vi "Save MES errors.vi"(9 "Sent parameters":variant, 10 "Error Text":string, 11 "Operation":string) -> ()   [LabVIEW 2023]
uses:
  <vilib>/Utility/file.llb/Write Delimited Spreadsheet (string).vi
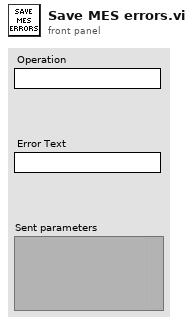
[diagram p1: front panel]
types:
  T1 = cluster{"MaterialCode":string, "Operator":string, "SerialNo":string}
  T2 = cluster{"HuNo":string, "MaterialCode":string, "Mode":i32, "Operator":string, "PackingInstructions":string, "ProductionVersion":string, "SerialNo":string}
  T3 = cluster{"EquipmentCode":string, "Mode":i32, "Operator":string}
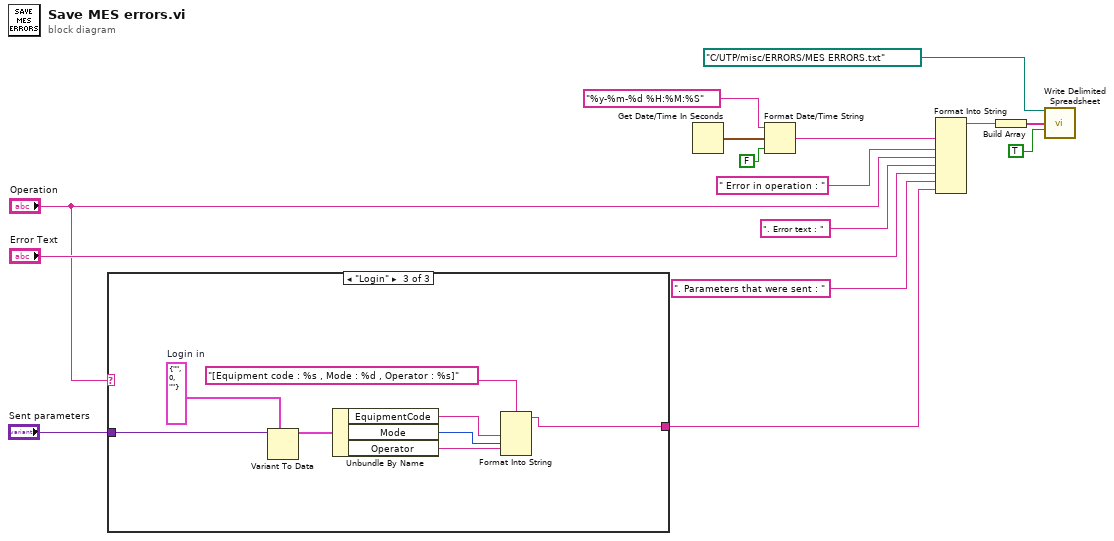
[diagram p0: block diagram]
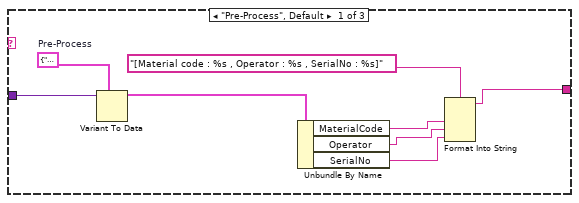
[diagram p2: hidden frame]
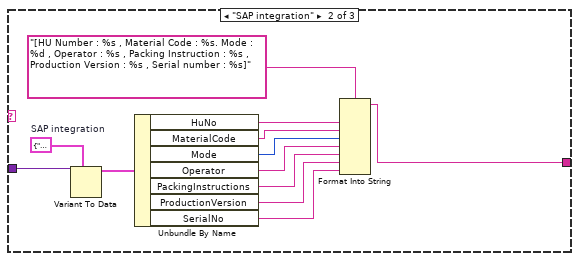
[diagram p3: hidden frame]
diagram:
  n1 = case shown="\"Login\"" "Operation" {
    tunnel: "Sent parameters" -> [w16 w35 w43]
    tunnel: [w18 w25 w36] -> w1
    frame "Pre-Process", Default {
      w17 = T1 {"MaterialCode"="", "Operator"="", "SerialNo"=""}  # Pre-Process
      n2 = Variant To Data(type=w17, Variant=w16) -> (data=w20:T1)  [unwired: 1 in, 1 out]
      n3 = Unbundle By Name(w20) -> ("MaterialCode"=w21:string, "Operator"=w22:string, "SerialNo"=w23:string)
      n4 = Format Into String(format string="[Material code : %s , Operator : %s , SerialNo : %s]", w21, w22, w23) -> (resulting string=w18:string)  [unwired: 2 in, 1 out]
    }
    frame "SAP integration" {
      w34 = T2 {"HuNo"="", "MaterialCode"="", "Mode"=0, "Operator"="", "PackingInstructions"="", "ProductionVersion"="", "SerialNo"=""}  # SAP integration
      n5 = Variant To Data(type=w34, Variant=w35) -> (data=w33:T2)  [unwired: 1 in, 1 out]
      n6 = Unbundle By Name(w33) -> ("HuNo"=w32:string, "MaterialCode"=w31:string, "Mode"=w30:i32, "Operator"=w29:string, "PackingInstructions"=w28:string, "ProductionVersion"=w27:string, "SerialNo"=w26:string)
      n7 = Format Into String(format string="[HU Number : %s , Material Code : %s. Mode : %d , Operator : %s , Packing Instruction : %s , Production Version : %s , Serial number : %s]", w32, w31, w30, w29, w28, w27, w26) -> (resulting string=w25:string)  [unwired: 2 in, 1 out]
    }
    frame "Login" {
      w42 = T3 {"EquipmentCode"="", "Mode"=0, "Operator"=""}  # Login in
      n8 = Variant To Data(type=w42, Variant=w43) -> (data=w41:T3)  [unwired: 1 in, 1 out]
      n9 = Unbundle By Name(w41) -> ("EquipmentCode"=w40:string, "Mode"=w39:i32, "Operator"=w38:string)
      n10 = Format Into String(format string="[Equipment code : %s , Mode : %d , Operator : %s]", w40, w39, w38) -> (resulting string=w36:string)  [unwired: 2 in, 1 out]
    }
  }
  n11 = Get Date/Time In Seconds() -> (seconds since 1Jan1904=w12:timestamp)
  n12 = Format Date/Time String(time format string (%c)="%y-%m-%d %H:%M:%S", seconds (now)=w12, UTC format=FALSE) -> (date/time string=w9:string)
  n13 = Format Into String(w9, " Error in operation : " ("input 2"), "Operation", ". Error text : " ("input 2"), "Error Text", ". Parameters that were sent : " ("input 2"), w1) -> (resulting string=w4:string)  [unwired: 3 in, 1 out]
  n14 = Build Array(w4) -> (w13:string[])
  n15 = call-poly <vilib>:"Write Delimited Spreadsheet.vi"("file path (dialog if empty)"=path "C:/UTP/misc/ERRORS/MES ERRORS.txt", "1D data"=w13, "append to file? (new file:F)"=TRUE) -> ()  [unwired: 11 in, 2 out]
